vi "Read Roles.vi"(8 "error in (no error)":errorcluster, 11 "PrepareFourthPassPlay in":refnum<class "PrepareFourthPassPlay.lvclass">) -> (0 "error out":errorcluster, 2 "Roles":T1, 3 "PrepareFourthPassPlay out":refnum<class "PrepareFourthPassPlay.lvclass">)   [LabVIEW 2020, in "PrepareFourthPassPlay.lvclass"]
uses:
  PrepareFourthPassPlay.lvclass
  PreparePassReceiverRole_class/PreparePassReceiverRole.lvclass
  AttackerStopRole_class/AttackerStopRole.lvclass
  PrepareFourthPassPlay.lvclass/PrepareFourthPassPlay.ctl
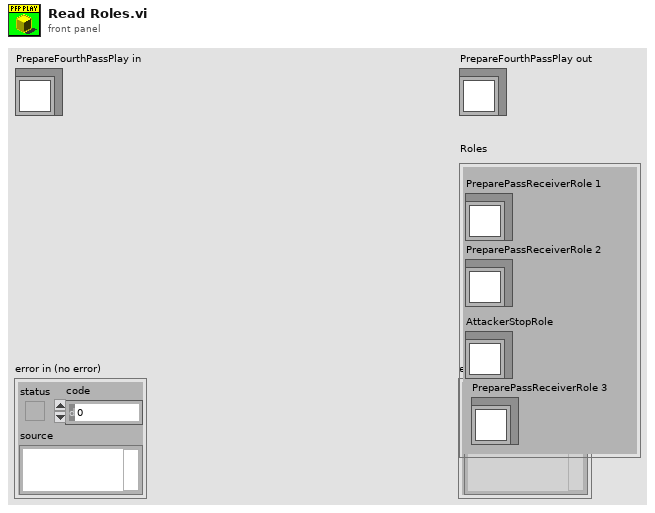
[diagram p1: front panel]
types:
  T1 = cluster{"PreparePassReceiverRole 1":refnum<class "PreparePassReceiverRole.lvclass">, "AttackerStopRole":refnum<class "AttackerStopRole.lvclass">, "PreparePassReceiverRole 2":refnum<class "PreparePassReceiverRole.lvclass">, "PreparePassReceiverRole 3":refnum<class "PreparePassReceiverRole.lvclass">}
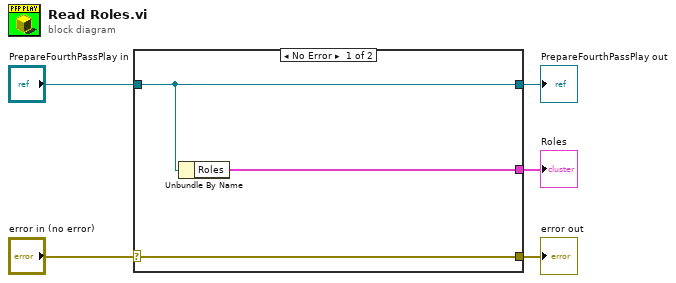
[diagram p0: block diagram]
diagram:
  n1 = case shown="No Error" "error in (no error)" {
    selector: "error in (no error)" -> [w8 w9]
    tunnel: [w8 w9] -> w4
    tunnel: [w7 w10] -> w2
    tunnel: "PrepareFourthPassPlay in" -> [w7 w10]
    tunnel: [w6 _] -> w1
    frame No Error {
      n2 = Unbundle By Name(w7) -> ("Roles"=w6:T1)
    }
    frame Error {
    }
  }
  "error out" <- w4
  "PrepareFourthPassPlay out" <- w2
  "Roles" <- w1
